vi "EnQ State.vi"(8 "error in (no error)":errorcluster, 10 "BitField":u16, 11 "Valve in":refnum<class "Valve.lvclass">) -> (0 "error out":errorcluster, 3 "Valve out":refnum<class "Valve.lvclass">)   [LabVIEW 2015, in "cRIO-Carbondioxide.lvlib" / "CO2-Actor.lvlib" / "Valve.lvclass"]
uses:
  Valve.lvclass
  Valve.lvclass/Valve.ctl
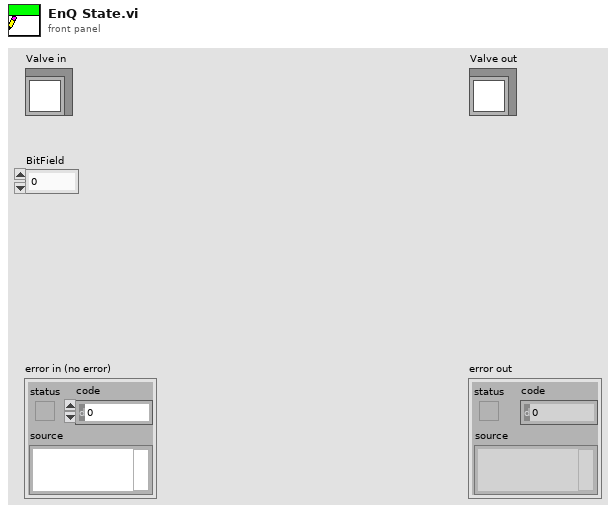
[diagram p1: front panel]
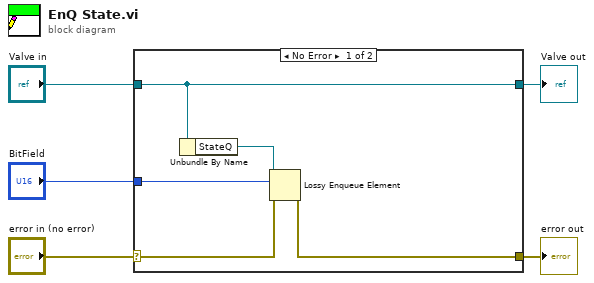
[diagram p0: block diagram]
diagram:
  n1 = case shown="No Error" "error in (no error)" {
    selector: "error in (no error)" -> [w9 w11]
    tunnel: [w8 w11] -> w4
    tunnel: [w7 w12] -> w2
    tunnel: "Valve in" -> [w7 w12]
    tunnel: "BitField" -> [w6 _]
    frame No Error {
      n2 = Unbundle By Name(w7) -> ("StateQ"=w10:refnum<queue>)
      n3 = Lossy Enqueue Element(queue=w10, element=w6, error in (no error)=w9) -> (error out=w8:errorcluster)  [unwired: 3 out]
    }
    frame Error {
    }
  }
  "error out" <- w4
  "Valve out" <- w2
